vi "Compare Var.vi"(5 "Value 1":variant caption="Value 1 (variant)", 9 "Value 2":variant caption="Value 2 (variant)", 11 "error in":errorcluster caption="error in (no error)") -> (8 "Equal?":bool, 15 "error out":errorcluster)   [LabVIEW 2014]
uses:
  <vilib>/Utility/VariantDataType/RefnumType.ctl
  <vilib>/Utility/VariantDataType/Type.ctl
  <vilib>/Utility/VariantDataType/VariantType.lvlib
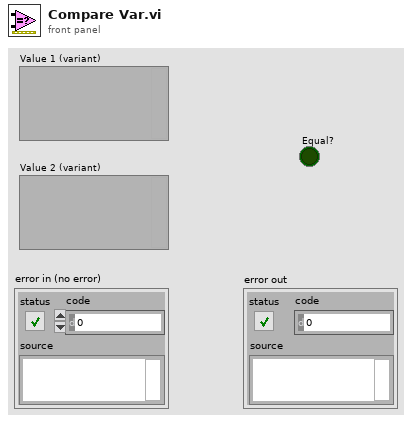
[diagram p1: front panel]
types:
  T1 = typedef "Type Descriptor Enumeration__ogtk.ctl" = enum8{"<Null>", "I8", "I16", "I32", "I64", "U8", "U16", "U32", "U64", "SGL", "DBL", "EXT", "CSG", "CDB", "CXT", "0x0F", "0x10", "0x11", "0x12", "0x13", "0x14", "Enum U8", "Enum U16", "Enum U32", "Enum U64", "SGL PQ", "DBL PQ", "EXT PQ", "CSG PQ", "CDB PQ", "CXT PQ", "0x1F", "0x20", "Boolean", "0x22", "0x23", "0x24", "0x25", "0x26", "0x27", "0x28", "0x29", "0x2A", "0x2B", "0x2C", "0x2D", "0x2E", "0x2F", "String", "0x31", "Path", "Pict", "0x34", "0x35", "0x36", "DAQ", "0x38", "0x39", "0x3A", "0x3B", "0x3C", "0x3D", "0x3E", "0x3F", "Array", "0x41", "0x42", "0x43", "0x44", "0x45", "0x46", "0x47", "0x48", "0x49", "0x4A", "0x4B", "0x4C", "0x4D", "0x4E", "0x4F", "Cluster", "0x51", "0x52", "Variant", "Waveform", "0x55", "0x56", "0x57", "0x58", "0x59", "0x5A", "0x5B", "0x5C", "0x5D", "0x5E", "0x5F", "0x60", "0x61", "0x62", "0x63", "0x64", "0x65", "0x66", "0x67", "0x68", "0x69", "0x6A", "0x6B", "0x6C", "0x6D", "0x6E", "0x6F", "Refnum"}
  T2 = typedef "VariantType.lvlib/RefnumType.ctl" = enum16{"NotARefnum", "UnknownRefnum", "Generic", "Datalog", "ByteStream", "Device", "Occurence", "TCPNetConnection", "Auto", "Menu", "Imaq", "Hardware", "DataSocket", "Visa", "IVI", "UDPNetConnection", "Notifier", "Queue", "Irda", "EventReg", "DotNet", "UserEvent", "Callback", "UNUSED_EMPTY_POSITION", "BlueToothNetConnection", "LVObjApp", "LVObjVI", "LVObjUnknown", "GenericClass", "UserDefinedRefnumTag", "DataValue", "RT FIFO", "TDMS File"}
  T3 = typedef "VariantType.lvlib/Type.ctl" = enum8{"Invalid Type", "Void", "I8", "I16", "I32", "I64", "U8", "U16", "U32", "U64", "Single Float", "Double Float", "Extended Float", "Single Complex", "Double Complex", "Extended Complex", "Enum U8", "Enum U16", "Enum U32", "Enum U64", "Single Float With Unit", "Double Float With Unit", "Extended Float With Unit", "Single Complex with Unit", "Double Complex with Unit", "Extended Complex with Unit", "Boolean", "String", "Path", "Picture", "Tag", "Array", "Cluster", "Variant", "LV Variant", "Waveform", "Timestamp", "Digital Waveform", "Digital Data", "ExpressData", "Refnum", "External Data", "VI", "Poly VI", "LabVIEW Class Instance", "Fixed Point"}
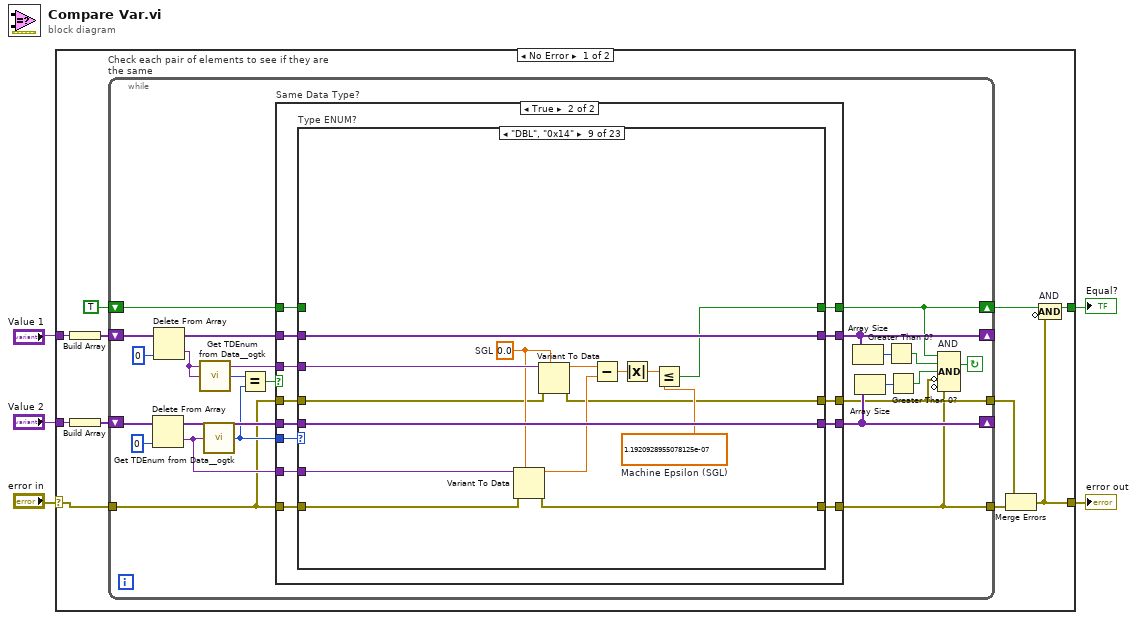
[diagram p0: block diagram]
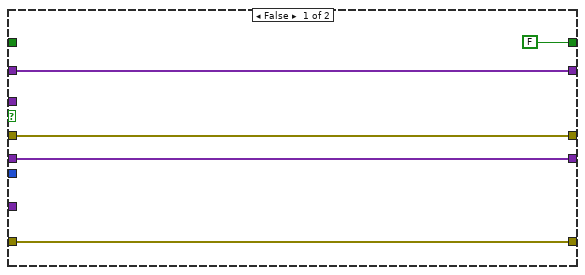
[diagram p2: hidden frame]
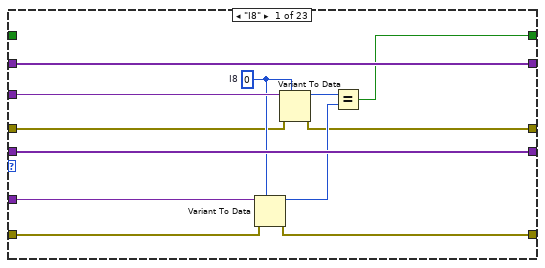
[diagram p3: hidden frame]
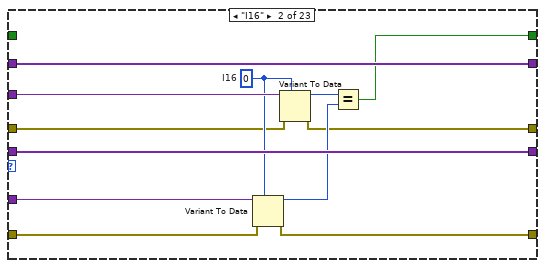
[diagram p4: hidden frame]
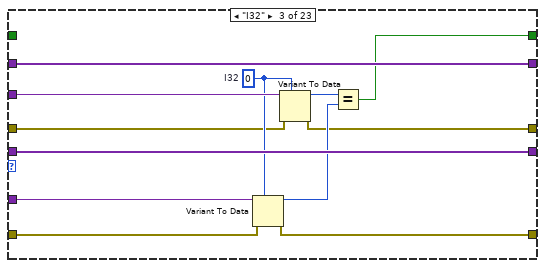
[diagram p5: hidden frame]
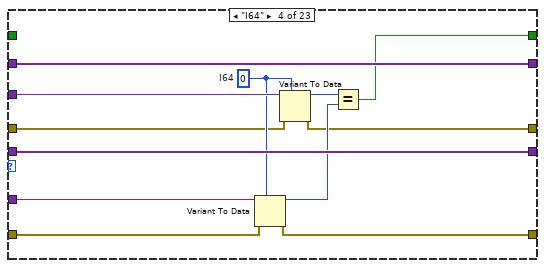
[diagram p6: hidden frame]
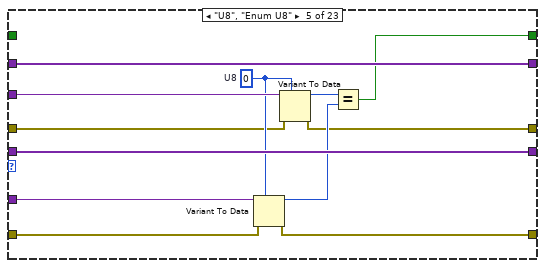
[diagram p7: hidden frame]
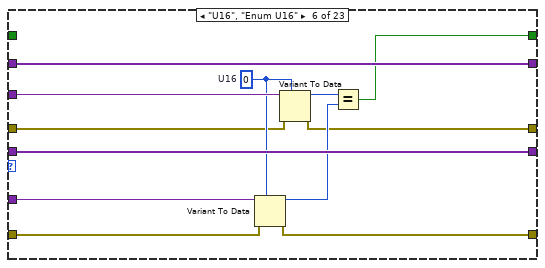
[diagram p8: hidden frame]
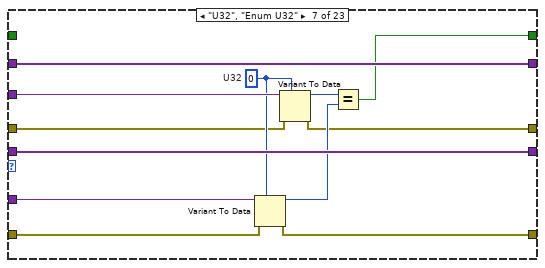
[diagram p9: hidden frame]
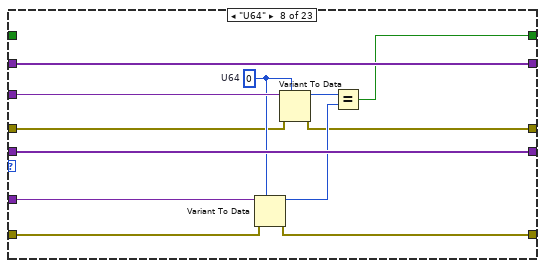
[diagram p10: hidden frame]
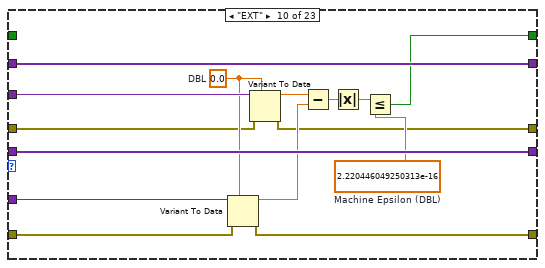
[diagram p11: hidden frame]
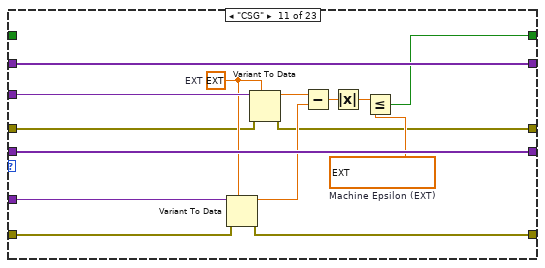
[diagram p12: hidden frame]
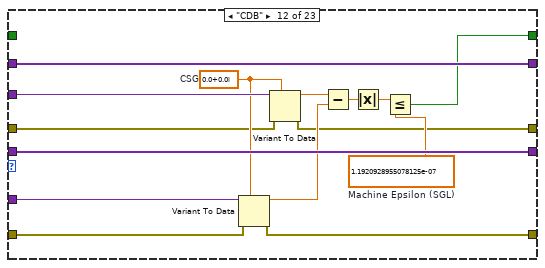
[diagram p13: hidden frame]
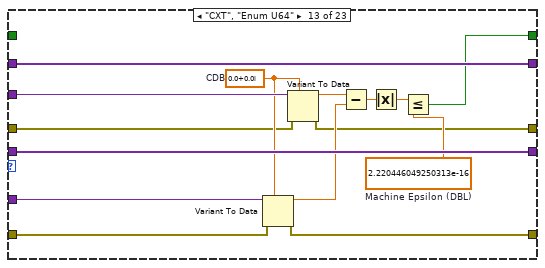
[diagram p14: hidden frame]
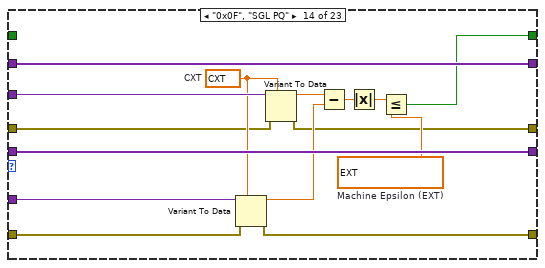
[diagram p15: hidden frame]
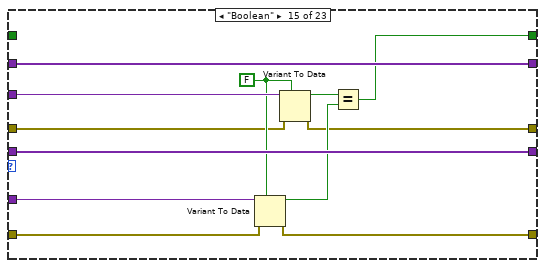
[diagram p16: hidden frame]
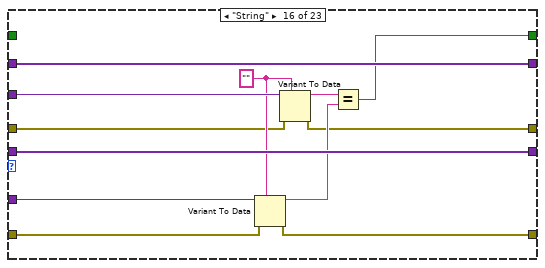
[diagram p17: hidden frame]
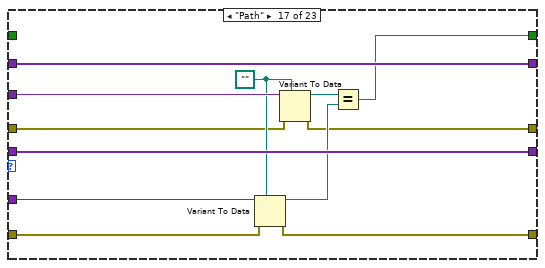
[diagram p18: hidden frame]
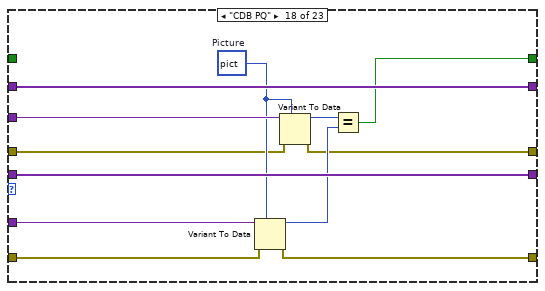
[diagram p19: hidden frame]
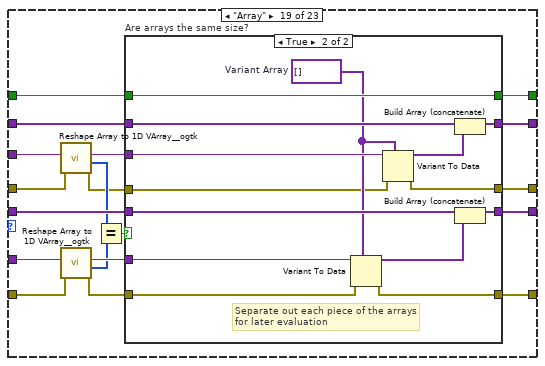
[diagram p20: hidden frame]
diagram:
  n1 = case shown="No Error" "error in" {
    selector: "error in" -> [w6 w411]
    tunnel: "Value 2" -> [w16 _]
    tunnel: "Value 1" -> [w14 _]
    tunnel: [w7 FALSE] -> w3
    tunnel: [w9 w411] -> w2
    frame No Error {
      n2 = Build Array(w14) -> (w13:variant[])
      n3 = Build Array(w16) -> (w15:variant[])
      n4 = while "Check each pair of elements to see if they are the same" {
        shift-right: [w35] -> _
        shift-left: w15 -> [w39]
        shift-right: [w25] -> w8
        shift-left: TRUE -> [w30]
        shift-right: [w28] -> _
        shift-left: w13 -> [w34]
        tunnel: [w23] -> w11
        tunnel: [w22] -> w10
        tunnel: w6 -> [w17]
        stop <- w24 continue-if-true
        n5 = Delete From Array(array=w39, index=0) -> (deleted portion=w19:variant, array with subset deleted=w36:variant[])  [unwired: 1 in]
        n6 = Delete From Array(array=w34, index=0) -> (deleted portion=w21:variant, array with subset deleted=w32:variant[])  [unwired: 1 in]
        n7 = call <userlib>:"Get TDEnum from Data__ogtk.vi"("Data"=w21) -> ("Type Descriptor Enumeration"=w20:T1)  [unwired: 4 in]
        n8 = call <userlib>:"Get TDEnum from Data__ogtk.vi"("Data"=w19) -> ("Type Descriptor Enumeration"=w18:T1)  [unwired: 4 in]
        n9 = Equal?(x=w20, y=w18) -> (x = y?=w31:bool)
        n10 = case "Same Data Type?" shown="True" w31 {
          tunnel: w19 -> [_ w57]
          tunnel: w36 -> [w42 w56]
          tunnel: [w42 w55] -> w35
          tunnel: w18 -> [_ w54]
          tunnel: w32 -> [w43 w53]
          tunnel: w21 -> [_ w52]
          tunnel: [w43 w51] -> w28
          tunnel: w30 -> [_ w50]
          tunnel: [FALSE w49] -> w25
          tunnel: w17 -> [w41 w48]
          tunnel: w17 -> [w40 w47]
          tunnel: [w41 w45] -> w23
          tunnel: [w40 w46] -> w22
          frame False {
          }
          frame True {
            n11 = case "Type ENUM?" shown="\"DBL\", \"0x14\"" w54 {
              tunnel: w57 -> [w67 w79 w91 w103 w115 w127 w139 w151 w166 w181 w196 w211 w226 w241 w253 w265 w277 w289 w303 w337 w352 w361 w405]
              tunnel: w56 -> [w68 w80 w92 w104 w116 w128 w140 w152 w167 w182 w197 w212 w227 w242 w254 w266 w278 w290 w310 w342 w353 w355 w408]
              tunnel: [w68 w80 w92 w104 w116 w128 w140 w152 w167 w182 w197 w212 w227 w242 w254 w266 w278 w290 w309 w341 w353 w355 w408] -> w55
              tunnel: w53 -> [w69 w81 w93 w105 w117 w129 w141 w153 w168 w183 w198 w213 w228 w243 w255 w267 w279 w291 w308 w340 w354 w356 w409]
              tunnel: w52 -> [w66 w78 w90 w102 w114 w126 w138 w150 w165 w180 w195 w210 w225 w240 w252 w264 w276 w288 w304 w335 w351 w363 w406]
              tunnel: [w69 w81 w93 w105 w117 w129 w141 w153 w168 w183 w198 w213 w228 w243 w255 w267 w279 w291 w307 w339 w354 w356 w409] -> w51
              tunnel: w50 -> [_ _ _ _ _ _ _ _ _ _ _ _ _ _ _ _ _ _ w306 w338 _ _ _]
              tunnel: [w62 w74 w86 w98 w110 w122 w134 w146 w158 w173 w188 w203 w218 w233 w248 w260 w272 w285 w305 w338 w348 w368 w407] -> w49
              tunnel: w48 -> [w60 w73 w85 w97 w109 w121 w133 w145 w157 w172 w186 w202 w217 w232 w247 w259 w271 w283 w302 w333 w346 w364 w404]
              tunnel: w47 -> [w61 w71 w83 w95 w107 w119 w131 w143 w155 w170 w187 w201 w216 w230 w245 w257 w269 w282 w301 w332 w345 w362 w403]
              tunnel: [w58 w70 w82 w94 w106 w118 w130 w142 w154 w169 w184 w200 w215 w229 w244 w256 w268 w281 w299 w330 w343 w366 w403] -> w46
              tunnel: [w59 w72 w84 w96 w108 w120 w132 w144 w156 w171 w185 w199 w214 w231 w246 w258 w270 w280 w300 w331 w344 w367 w404] -> w45
              frame "I8" {
                w65 = i8 0  # I8
                n12 = Variant To Data(error in=w61, type=w65, Variant=w67) -> (data=w63:i8, error out=w58:errorcluster)
                n13 = Variant To Data(error in=w60, type=w65, Variant=w66) -> (data=w64:i8, error out=w59:errorcluster)
                n14 = Equal?(x=w64, y=w63) -> (x = y?=w62:bool)
              }
              frame "I16" {
                w77 = i16 0  # I16
                n15 = Variant To Data(error in=w71, type=w77, Variant=w79) -> (data=w75:i16, error out=w70:errorcluster)
                n16 = Variant To Data(error in=w73, type=w77, Variant=w78) -> (data=w76:i16, error out=w72:errorcluster)
                n17 = Equal?(x=w76, y=w75) -> (x = y?=w74:bool)
              }
              frame "I32" {
                w89 = 0  # I32
                n18 = Variant To Data(error in=w83, type=w89, Variant=w91) -> (data=w87:i32, error out=w82:errorcluster)
                n19 = Variant To Data(error in=w85, type=w89, Variant=w90) -> (data=w88:i32, error out=w84:errorcluster)
                n20 = Equal?(x=w88, y=w87) -> (x = y?=w86:bool)
              }
              frame "I64" {
                w101 = i64 0  # I64
                n21 = Variant To Data(error in=w95, type=w101, Variant=w103) -> (data=w99:i64, error out=w94:errorcluster)
                n22 = Variant To Data(error in=w97, type=w101, Variant=w102) -> (data=w100:i64, error out=w96:errorcluster)
                n23 = Equal?(x=w100, y=w99) -> (x = y?=w98:bool)
              }
              frame "U8", "Enum U8" {
                w113 = u8 0  # U8
                n24 = Variant To Data(error in=w107, type=w113, Variant=w115) -> (data=w111:u8, error out=w106:errorcluster)
                n25 = Variant To Data(error in=w109, type=w113, Variant=w114) -> (data=w112:u8, error out=w108:errorcluster)
                n26 = Equal?(x=w112, y=w111) -> (x = y?=w110:bool)
              }
              frame "U16", "Enum U16" {
                w125 = u16 0  # U16
                n27 = Variant To Data(error in=w119, type=w125, Variant=w127) -> (data=w123:u16, error out=w118:errorcluster)
                n28 = Variant To Data(error in=w121, type=w125, Variant=w126) -> (data=w124:u16, error out=w120:errorcluster)
                n29 = Equal?(x=w124, y=w123) -> (x = y?=w122:bool)
              }
              frame "U32", "Enum U32" {
                w137 = u32 0  # U32
                n30 = Variant To Data(error in=w131, type=w137, Variant=w139) -> (data=w135:u32, error out=w130:errorcluster)
                n31 = Variant To Data(error in=w133, type=w137, Variant=w138) -> (data=w136:u32, error out=w132:errorcluster)
                n32 = Equal?(x=w136, y=w135) -> (x = y?=w134:bool)
              }
              frame "U64" {
                w149 = u64 0  # U64
                n33 = Variant To Data(error in=w143, type=w149, Variant=w151) -> (data=w147:u64, error out=w142:errorcluster)
                n34 = Variant To Data(error in=w145, type=w149, Variant=w150) -> (data=w148:u64, error out=w144:errorcluster)
                n35 = Equal?(x=w148, y=w147) -> (x = y?=w146:bool)
              }
              frame "DBL", "0x14" {
                w159 = sgl 1.1920929e-07  # Machine Epsilon (SGL)
                w164 = sgl 0.0  # SGL
                n36 = Variant To Data(error in=w155, type=w164, Variant=w166) -> (data=w162:sgl, error out=w154:errorcluster)
                n37 = Variant To Data(error in=w157, type=w164, Variant=w165) -> (data=w163:sgl, error out=w156:errorcluster)
                n38 = Subtract(x=w163, y=w162) -> (x-y=w161:sgl)
                n39 = Absolute Value(x=w161) -> (abs(x)=w160:sgl)
                n40 = Less Or Equal?(x=w160, y=w159) -> (x <= y?=w158:bool)
              }
              frame "EXT" {
                w174 = 2.220446049250313e-16  # Machine Epsilon (DBL)
                w179 = 0.0  # DBL
                n41 = Variant To Data(error in=w170, type=w179, Variant=w181) -> (data=w177:dbl, error out=w169:errorcluster)
                n42 = Variant To Data(error in=w172, type=w179, Variant=w180) -> (data=w178:dbl, error out=w171:errorcluster)
                n43 = Subtract(x=w178, y=w177) -> (x-y=w176:dbl)
                n44 = Absolute Value(x=w176) -> (abs(x)=w175:dbl)
                n45 = Less Or Equal?(x=w175, y=w174) -> (x <= y?=w173:bool)
              }
              frame "CSG" {
                w189 = ext 1.0842021724855044e-19  # Machine Epsilon (EXT)
                w194 = ext 0.0  # EXT
                n46 = Variant To Data(error in=w187, type=w194, Variant=w196) -> (data=w192:ext, error out=w184:errorcluster)
                n47 = Variant To Data(error in=w186, type=w194, Variant=w195) -> (data=w193:ext, error out=w185:errorcluster)
                n48 = Subtract(x=w193, y=w192) -> (x-y=w191:ext)
                n49 = Absolute Value(x=w191) -> (abs(x)=w190:ext)
                n50 = Less Or Equal?(x=w190, y=w189) -> (x <= y?=w188:bool)
              }
              frame "CDB" {
                w204 = sgl 1.1920929e-07  # Machine Epsilon (SGL)
                w209 = csg 0.0+0.0i  # CSG
                n51 = Variant To Data(error in=w201, type=w209, Variant=w211) -> (data=w207:csg, error out=w200:errorcluster)
                n52 = Variant To Data(error in=w202, type=w209, Variant=w210) -> (data=w208:csg, error out=w199:errorcluster)
                n53 = Subtract(x=w208, y=w207) -> (x-y=w206:csg)
                n54 = Absolute Value(x=w206) -> (abs(x)=w205:sgl)
                n55 = Less Or Equal?(x=w205, y=w204) -> (x <= y?=w203:bool)
              }
              frame "CXT", "Enum U64" {
                w219 = 2.220446049250313e-16  # Machine Epsilon (DBL)
                w224 = cdb 0.0+0.0i  # CDB
                n56 = Variant To Data(error in=w216, type=w224, Variant=w226) -> (data=w222:cdb, error out=w215:errorcluster)
                n57 = Variant To Data(error in=w217, type=w224, Variant=w225) -> (data=w223:cdb, error out=w214:errorcluster)
                n58 = Subtract(x=w223, y=w222) -> (x-y=w221:cdb)
                n59 = Absolute Value(x=w221) -> (abs(x)=w220:dbl)
                n60 = Less Or Equal?(x=w220, y=w219) -> (x <= y?=w218:bool)
              }
              frame "0x0F", "SGL PQ" {
                w234 = ext 1.0842021724855044e-19  # Machine Epsilon (EXT)
                w239 = cxt 0.0+0.0i  # CXT
                n61 = Variant To Data(error in=w230, type=w239, Variant=w241) -> (data=w237:cxt, error out=w229:errorcluster)
                n62 = Variant To Data(error in=w232, type=w239, Variant=w240) -> (data=w238:cxt, error out=w231:errorcluster)
                n63 = Subtract(x=w238, y=w237) -> (x-y=w236:cxt)
                n64 = Absolute Value(x=w236) -> (abs(x)=w235:ext)
                n65 = Less Or Equal?(x=w235, y=w234) -> (x <= y?=w233:bool)
              }
              frame "Boolean" {
                w251 = FALSE
                n66 = Variant To Data(error in=w245, type=w251, Variant=w253) -> (data=w249:bool, error out=w244:errorcluster)
                n67 = Variant To Data(error in=w247, type=w251, Variant=w252) -> (data=w250:bool, error out=w246:errorcluster)
                n68 = Equal?(x=w250, y=w249) -> (x = y?=w248:bool)
              }
              frame "String" {
                w263 = ""
                n69 = Variant To Data(error in=w257, type=w263, Variant=w265) -> (data=w261:string, error out=w256:errorcluster)
                n70 = Variant To Data(error in=w259, type=w263, Variant=w264) -> (data=w262:string, error out=w258:errorcluster)
                n71 = Equal?(x=w262, y=w261) -> (x = y?=w260:bool)
              }
              frame "Path" {
                w275 = path ""
                n72 = Variant To Data(error in=w269, type=w275, Variant=w277) -> (data=w273:path, error out=w268:errorcluster)
                n73 = Variant To Data(error in=w271, type=w275, Variant=w276) -> (data=w274:path, error out=w270:errorcluster)
                n74 = Equal?(x=w274, y=w273) -> (x = y?=w272:bool)
              }
              frame "CDB PQ" {
                w284 = picture data[5B]  # Picture
                n75 = Variant To Data(error in=w282, type=w284, Variant=w289) -> (data=w286:picture, error out=w281:errorcluster)
                n76 = Variant To Data(error in=w283, type=w284, Variant=w288) -> (data=w287:picture, error out=w280:errorcluster)
                n77 = Equal?(x=w287, y=w286) -> (x = y?=w285:bool)
              }
              frame "Array" {
                n78 = call <userlib>:"Reshape Array to 1D VArray__ogtk.vi"("error in (no error)"=w302, "MultiD Array"=w304) -> ("error out"=w293:errorcluster, "Size(s)"=w294:u32[], "1D VArray"=w297:variant)  [unwired: 7 in]
                n79 = call <userlib>:"Reshape Array to 1D VArray__ogtk.vi"("error in (no error)"=w301, "MultiD Array"=w303) -> ("error out"=w292:errorcluster, "Size(s)"=w295:u32[], "1D VArray"=w296:variant)  [unwired: 7 in]
                n80 = Equal?(x=w294, y=w295) -> (x = y?=w298:bool)
                n81 = case "Are arrays the same size?" shown="True" w298 {
                  tunnel: w310 -> [w313 w329]
                  tunnel: [w313 w328] -> w309
                  tunnel: w308 -> [w314 w327]
                  tunnel: [w314 w326] -> w307
                  tunnel: w306 -> [_ w325]
                  tunnel: [FALSE w325] -> w305
                  tunnel: w297 -> [_ w322]
                  tunnel: w296 -> [_ w324]
                  tunnel: w293 -> [w312 w319]
                  tunnel: w292 -> [w311 w318]
                  tunnel: [w312 w317] -> w300
                  tunnel: [w311 w316] -> w299
                  frame False {
                  }
                  frame True {
                    w320 = variant[] []  # Variant Array
                    # "Separate out each piece of the arrays\nfor later evaluation"
                    n82 = Variant To Data(error in=w318, type=w320, Variant=w324) -> (data=w323:variant[], error out=w316:errorcluster)
                    n83 = Variant To Data(error in=w319, type=w320, Variant=w322) -> (data=w321:variant[], error out=w317:errorcluster)
                    n84 = Build Array (concatenate)(w327, w321) -> (w326:variant[])
                    n85 = Build Array (concatenate)(w329, w323) -> (w328:variant[])
                  }
                }
              }
              frame "Cluster" {
                n86 = call <userlib>:"Cluster to Array of VData__ogtk.vi"("error in (no error)"=w332, "Cluster"=w337) -> ("error out"=w330:errorcluster, "Array of VData"=w336:variant[])  [unwired: 8 in]
                n87 = call <userlib>:"Cluster to Array of VData__ogtk.vi"("error in (no error)"=w333, "Cluster"=w335) -> ("error out"=w331:errorcluster, "Array of VData"=w334:variant[])  [unwired: 8 in]
                n88 = Build Array (concatenate)(w340, w334) -> (w339:variant[])
                n89 = Build Array (concatenate)(w342, w336) -> (w341:variant[])
              }
              frame "0x24" {
                w347 = timestamp(0 s since 1904-01-01)  # Timestamp
                n90 = Variant To Data(error in=w345, type=w347, Variant=w352) -> (data=w349:timestamp, error out=w343:errorcluster)
                n91 = Variant To Data(error in=w346, type=w347, Variant=w351) -> (data=w350:timestamp, error out=w344:errorcluster)
                n92 = Equal?(x=w350, y=w349) -> (x = y?=w348:bool)
              }
              frame "Refnum" {
                n93 = call <vilib>:"GetRefnumInfo.vi"("error in (no error)"=w364, "Variant"=w363) -> ("error out"=w359:errorcluster, "ReferenceType"=w360:T2)  [unwired: 6 in, 2 out]
                n94 = call <vilib>:"GetRefnumInfo.vi"("error in (no error)"=w362, "Variant"=w361) -> ("error out"=w358:errorcluster, "ReferenceType"=w357:T2)  [unwired: 6 in, 2 out]
                n95 = Equal?(x=w360, y=w357) -> (x = y?=w365:bool)
                n96 = case "Same type of refnum?" shown="True" w365 {
                  tunnel: [FALSE w379] -> w368
                  tunnel: w359 -> [w371 w378]
                  tunnel: [w371 w377] -> w367
                  tunnel: w358 -> [w370 w376]
                  tunnel: [w370 w375] -> w366
                  tunnel: w363 -> [_ w374]
                  tunnel: w361 -> [_ w373]
                  tunnel: w357 -> [_ w372]
                  frame False {
                  }
                  frame True {
                    (unwired) RefnumType."NotARefnum"  # ReferenceTypes
                    n97 = case "Reference Type?" shown="Default" w372 {
                      tunnel: w374 -> [w389 w402]
                      tunnel: [w388 w401] -> w379
                      tunnel: w378 -> [w387 w400]
                      tunnel: [w386 w399] -> w377
                      tunnel: w376 -> [w385 w397]
                      tunnel: [w384 w396] -> w375
                      tunnel: w373 -> [w383 w398]
                      frame "Hardware", "Visa", "IVI" {
                        w380 = refnum<visa-resource-name> refnum ("VISA resource name")
                        n98 = Variant To Data(error in=w385, type=w380, Variant=w383) -> (data=w382:refnum<visa-resource-name>, error out=w384:errorcluster)
                        n99 = Variant To Data(error in=w387, type=w380, Variant=w389) -> (data=w381:refnum<visa-resource-name>, error out=w386:errorcluster)
                        n100 = Equal?(x=w381, y=w382) -> (x = y?=w388:bool)
                      }
                      frame Default {
                        w391 = 0  # I32
                        w394 = refnum<k0> refnum
                        # "This is a catch-all case for all the other refnums including those that defy predefinition because they reference and are typdef'd by a user defined data structure (e.g. notifiers, queues, datalog file reference, ...)"
                        n101 = Variant To Data(error in=w397, type=w394, Variant=w398) -> (data=w390:refnum<k0>, error out=w396:errorcluster)
                        n102 = Variant To Data(error in=w400, type=w394, Variant=w402) -> (data=w395:refnum<k0>, error out=w399:errorcluster)
                        n103 = Type Cast(type=w391, x=w395) -> (*(type *) &x=w393:i32)
                        n104 = Type Cast(type=w391, x=w390) -> (*(type *) &x=w392:i32)
                        n105 = Equal?(x=w393, y=w392) -> (x = y?=w401:bool)
                      }
                    }
                  }
                }
              }
              frame Default {
                (unwired) Type."LV Variant" ("NI \"Info\" Type Enum")
                (unwired) Type."Variant" ("NI \"Info\" Type Enum")
                (unwired) Type."Void" ("NI \"Info\" Type Enum")
                (unwired) Type."Invalid Type" ("NI \"Info\" Type Enum")
                (unwired) Type."Fixed Point" ("NI \"Info\" Type Enum")
                (unwired) Type."LabVIEW Class Instance" ("NI \"Info\" Type Enum")
                (unwired) Type."Poly VI" ("NI \"Info\" Type Enum")
                (unwired) Type."VI" ("NI \"Info\" Type Enum")
                (unwired) Type."External Data" ("NI \"Info\" Type Enum")
                (unwired) Type."ExpressData" ("NI \"Info\" Type Enum")
                (unwired) Type."Digital Data" ("NI \"Info\" Type Enum")
                (unwired) Type."Digital Waveform" ("NI \"Info\" Type Enum")
                (unwired) Type."Waveform" ("NI \"Info\" Type Enum")
                (unwired) Type."Tag" ("NI \"Info\" Type Enum")
                # "These types have not yet been explicitly handled in other cases"
                n106 = Equal?(x=w406, y=w405) -> (x = y?=w407:bool)
              }
            }
          }
        }
        n107 = Array Size(array=w28) -> (size(s)=w29:i32)
        n108 = Array Size(array=w35) -> (size(s)=w37:i32)
        n109 = Greater Than 0?(x=w29) -> (x > 0?=w26:bool)
        n110 = Greater Than 0?(x=w37) -> (x > 0?=w27:bool)
        n111 = Compound Arithmetic op=AND "AND"(w25, w26, w27, invert w23, invert w22) -> (w24:bool)
      }
      n112 = Merge Errors(w11, w10) -> (w9:errorcluster)
      n113 = Compound Arithmetic op=AND "AND"(w8, invert w9) -> (w7:bool)
    }
    frame Error {
    }
  }
  "Equal?" <- w3
  "error out" <- w2
